vi "detOf2x2.vi"(1 "2x2Matrix":dbl[][](array[numeric])) -> (0 "Determinant":dbl)   [LabVIEW 2015]
doc: "2x2Matrix -- It's a 2x2 array.\nDeterminant -- The determinant of the 2x2 Matrix(input)."
panel:
  in  "stop":bool
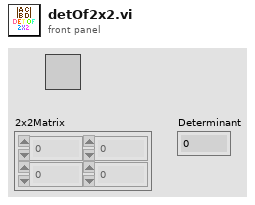
[diagram p1: front panel]
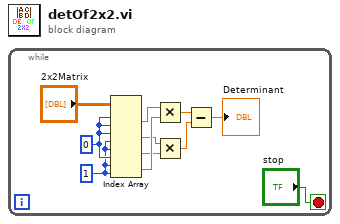
[diagram p0: block diagram]
diagram:
  n1 = while {
    stop <- "stop" stop-if-true
    w9 = 1 ("disabled index (col)")
    w10 = 0 ("index (row)")
    n2 = Index Array(array="2x2Matrix", index (row) #1=w10, index (col) #1=w10, index (row) #2=w10, index (col) #2=w9, index (row) #3=w9, index (col) #3=w10, index (row) #4=w9, index (col) #4=w9) -> (element #1=w8:dbl, element #2=w6:dbl, element #3=w5:dbl, element #4=w7:dbl)
    n3 = Multiply(x=w8, y=w7) -> (x*y=w4:dbl)
    n4 = Multiply(x=w6, y=w5) -> (x*y=w3:dbl)
    n5 = Subtract(x=w4, y=w3) -> (x-y=→"Determinant":dbl)
  }
